vi "State Seperator CONSTANT.vi"() -> (0 "Seperator (:)":string)   [LabVIEW 2011, in "State Machine Lib.lvlib"]
doc: "Used to build and parse state hierarchies."
uses:
  State Machine Lib.lvlib
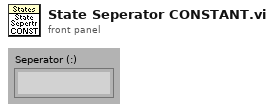
[diagram p1: front panel]
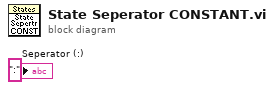
[diagram p0: block diagram]
diagram:
  "Seperator (:)" <- ":" ("regular expression")
